vi "Dataflow.vi"() -> ()   [LabVIEW 2014, in "LVOOP Introduction.lvlib"]
doc: "This VI is used to explain the dataflow paradigma.\n\nLizenziert unter EUPL V. 1.1"
uses:
  LVOOP Introduction.lvlib
panel:
  out "Result 2":dbl
  out "Result 1":dbl
  in  "Number":dbl
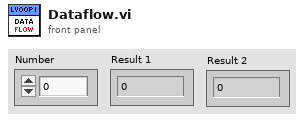
[diagram p1: front panel]
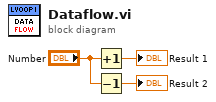
[diagram p0: block diagram]
diagram:
  n1 = Increment(x="Number") -> (x+1=→"Result 1":dbl)
  n2 = Decrement(x="Number") -> (x-1=→"Result 2":dbl)
